vi "GetShooterRefs.vi"(8 "error in (no error)":errorcluster) -> (0 "error out":errorcluster, 3 "cluster out":T17={"Shooter Ratchet"={"DevStatus"={"status"=FALSE, "code"=0, "source"=""}, "Solenoid Module"=enum."Solenoid Module 1", "Forward Solenoid Channel"=enum."Solenoid 1", "Reverse Solenoid Channel"=enum."Solenoid 1"}, "Shooter Limit"={"DevStatus"={"status"=FALSE, "code"=0, "source"=""}, "DIO Channel"=enum."DIO 1", "Digital Module"=enum."Digital Module 1"}, "Shooter Dog"={"DevStatus"={"status"=FALSE, "code"=0, "source"=""}, "Solenoid Module"=enum."Solenoid Module 1", "Forward Solenoid Channel"=enum."Solenoid 1", "Reverse Solenoid Channel"=enum."Solenoid 1"}, "Wipers"={"DevStatus"={"status"=FALSE, "code"=0, "source"=""}, "Solenoid Module"=enum."Solenoid Module 1", "Forward Solenoid Channel"=enum."Solenoid 1", "Reverse Solenoid Channel"=enum."Solenoid 1"}, "Winch"={"DeviceStatus"={"status"=FALSE, "code"=0, "source"=""}, "Type"=enum."PWM", "PWM"={"Digital Module"=enum."Digital Module 1", "PWM Channel"=enum."PWM 1", "DeadBand"={"Name"="", "maxPositivePwm"=0, "minPositivePwm"=0, "centerPwm"=0, "maxNegativePwm"=0, "minNegativePwm"=0, "angularRange"=0}}, "CAN"={"Device Number"=0, "Control Mode"=enum."Percent VBus", "Semaphore"=refnum, "Max Vout"=0.0}, "Invert"=FALSE, "TransformRef"=refnum, "InvTransformRef"=refnum}, "Hall"={"DevStatus"={"status"=FALSE, "code"=0, "source"=""}, "DIO Channel"=enum."Invalid", "Digital Module"=enum."Digital Module 1"}, "Catch"={"DevStatus"={"status"=FALSE, "code"=0, "source"=""}, "Solenoid Module"=enum."Solenoid Module 1", "Forward Solenoid Channel"=enum."Invalid", "Reverse Solenoid Channel"=enum."Invalid"}, "Compressor"={"DevStatus"={"status"=FALSE, "code"=0, "source"=""}, "DigitalInputDevRef"={"DevStatus"={"status"=FALSE, "code"=0, "source"=""}, "DIO Channel"=enum."DIO 1", "Digital Module"=enum."Digital Module 1"}, "RelayDevRef"={"DevStatus"={"status"=FALSE, "code"=0, "source"=""}, "Relay Channel"=enum."Invalid", "Digital Module"=enum."Digital Module 1", "Relay Direction"=enum."Both directions"}}})   [LabVIEW 2013]
uses:
  <vilib>/Rock Robotics/WPI/Solenoid/WPI_SolenoidDevRef.ctl
  <vilib>/Rock Robotics/SystemInterfaces/Typedef/FPGA_TypedefSolenoidModule.ctl
  <vilib>/Rock Robotics/WPI/Solenoid/WPI_SolenoidChannel.ctl
  <vilib>/Rock Robotics/WPI/DigitalInput/WPI_DigitalInputDevRef.ctl
  <vilib>/Rock Robotics/SystemInterfaces/DIO/FPGA_DIOChannel.ctl
  <vilib>/Rock Robotics/SystemInterfaces/Typedef/FPGA_TypedefDigitalModule.ctl
  <vilib>/Rock Robotics/WPI/MotorControl/WPI_MotorControlDeviceRef.ctl
  <vilib>/Rock Robotics/SystemInterfaces/DIO/FPGA_DIOPWMChannel.ctl
  <vilib>/Rock Robotics/WPI/PWM/WPI_PWMDeadband.ctl
  <vilib>/Rock Robotics/WPI/CAN/Jaguar/SubVIs/WPI_CANJaguar_ControlMode.ctl
  <vilib>/Rock Robotics/WPI/PWM/WPI_PWMTransform_ConPane.ctl
  <vilib>/Rock Robotics/WPI/Compressor/WPI_CompressorDevRef.ctl
  <vilib>/Rock Robotics/WPI/Relay/WPI_RelayDevRef.ctl
  <vilib>/Rock Robotics/SystemInterfaces/DIO/FPGA_DIORelayChannel.ctl
  <vilib>/Rock Robotics/WPI/Relay/WPI_RelayDirection.ctl
panel:
  in  "cluster in":T17={"Shooter Ratchet"={"DevStatus"={"status"=FALSE, "code"=0, "source"=""}, "Solenoid Module"=enum."Solenoid Module 1", "Forward Solenoid Channel"=enum."Solenoid 1", "Reverse Solenoid Channel"=enum."Solenoid 1"}, "Shooter Limit"={"DevStatus"={"status"=FALSE, "code"=0, "source"=""}, "DIO Channel"=enum."DIO 1", "Digital Module"=enum."Digital Module 1"}, "Shooter Dog"={"DevStatus"={"status"=FALSE, "code"=0, "source"=""}, "Solenoid Module"=enum."Solenoid Module 1", "Forward Solenoid Channel"=enum."Solenoid 1", "Reverse Solenoid Channel"=enum."Solenoid 1"}, "Wipers"={"DevStatus"={"status"=FALSE, "code"=0, "source"=""}, "Solenoid Module"=enum."Solenoid Module 1", "Forward Solenoid Channel"=enum."Solenoid 1", "Reverse Solenoid Channel"=enum."Solenoid 1"}, "Winch"={"DeviceStatus"={"status"=FALSE, "code"=0, "source"=""}, "Type"=enum."PWM", "PWM"={"Digital Module"=enum."Digital Module 1", "PWM Channel"=enum."PWM 1", "DeadBand"={"Name"="", "maxPositivePwm"=0, "minPositivePwm"=0, "centerPwm"=0, "maxNegativePwm"=0, "minNegativePwm"=0, "angularRange"=0}}, "CAN"={"Device Number"=0, "Control Mode"=enum."Percent VBus", "Semaphore"=refnum, "Max Vout"=0.0}, "Invert"=FALSE, "TransformRef"=refnum, "InvTransformRef"=refnum}, "Hall"={"DevStatus"={"status"=FALSE, "code"=0, "source"=""}, "DIO Channel"=enum."Invalid", "Digital Module"=enum."Digital Module 1"}, "Catch"={"DevStatus"={"status"=FALSE, "code"=0, "source"=""}, "Solenoid Module"=enum."Solenoid Module 1", "Forward Solenoid Channel"=enum."Invalid", "Reverse Solenoid Channel"=enum."Invalid"}, "Compressor"={"DevStatus"={"status"=FALSE, "code"=0, "source"=""}, "DigitalInputDevRef"={"DevStatus"={"status"=FALSE, "code"=0, "source"=""}, "DIO Channel"=enum."DIO 1", "Digital Module"=enum."Digital Module 1"}, "RelayDevRef"={"DevStatus"={"status"=FALSE, "code"=0, "source"=""}, "Relay Channel"=enum."Invalid", "Digital Module"=enum."Digital Module 1", "Relay Direction"=enum."Both directions"}}}
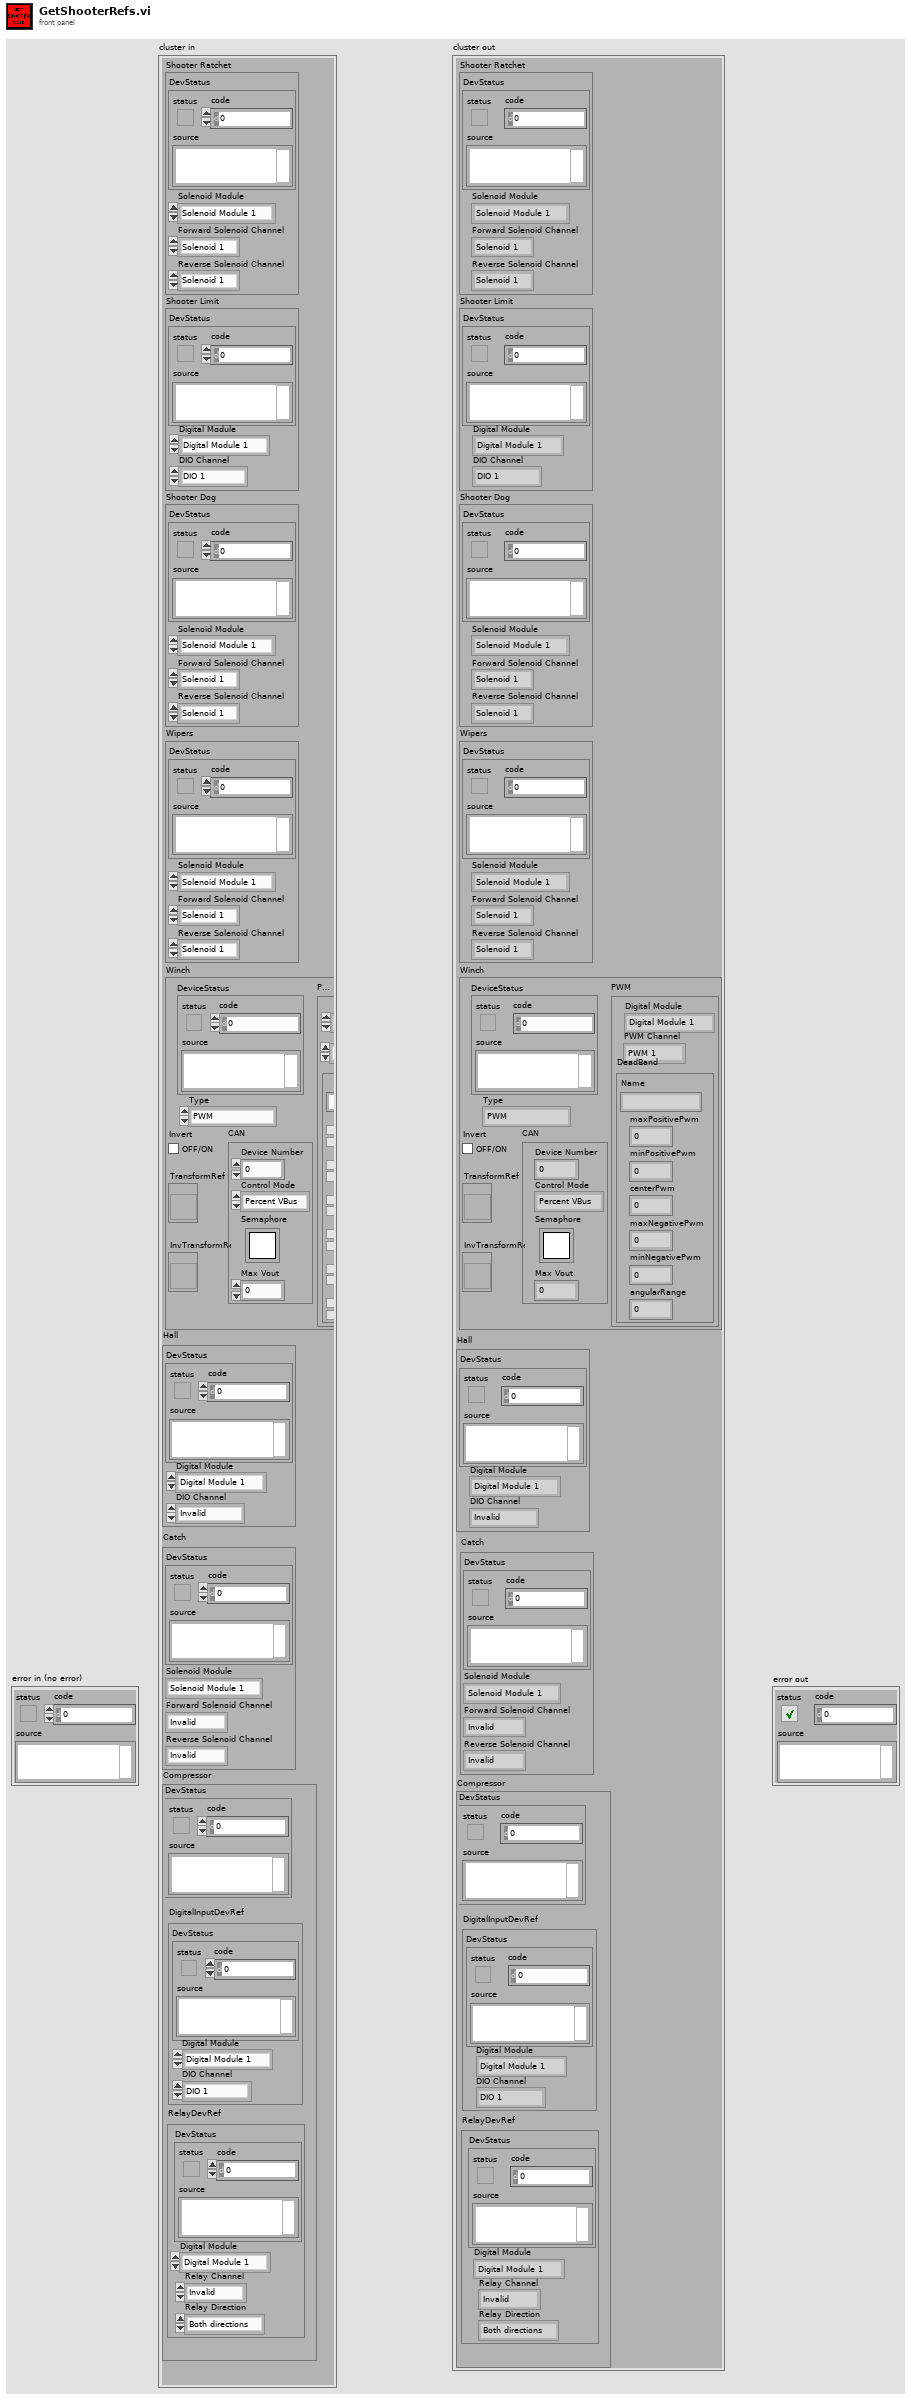
[diagram p1: front panel]
types:
  T1 = typedef "WPI_SolenoidDevRef.ctl" = cluster{"DevStatus":errorcluster, "Solenoid Module":T2, "Forward Solenoid Channel":T3, "Reverse Solenoid Channel":T3}
  T2 = typedef "FPGA_TypedefSolenoidModule.ctl" = enum16{"Solenoid Module 1", "Solenoid Module 2"}
  T3 = typedef "WPI_SolenoidChannel.ctl" = enum8{"Solenoid 1", "Solenoid 2", "Solenoid 3", "Solenoid 4", "Solenoid 5", "Solenoid 6", "Solenoid 7", "Solenoid 8", "Invalid"}
  T4 = typedef "WPI_DigitalInputDevRef.ctl" = cluster{"DevStatus":errorcluster, "DIO Channel":T5, "Digital Module":T6}
  T5 = typedef "FPGA_DIOChannel.ctl" = enum8{"DIO 1", "DIO 2", "DIO 3", "DIO 4", "DIO 5", "DIO 6", "DIO 7", "DIO 8", "DIO 9", "DIO 10", "DIO 11", "DIO 12", "DIO 13", "DIO 14", "Invalid"}
  T6 = typedef "FPGA_TypedefDigitalModule.ctl" = enum16{"Digital Module 1", "Digital Module 2"}
  T7 = typedef "WPI_MotorControlDeviceRef.ctl" = cluster{"DeviceStatus":errorcluster, "Type":enum16{"PWM", "CAN"}, "PWM":cluster{"Digital Module":T6, "PWM Channel":T8, "DeadBand":T9}, "CAN":cluster{"Device Number":u8, "Control Mode":T10, "Semaphore":T11, "Max Vout":dbl}, "Invert":bool, "TransformRef":T12, "InvTransformRef":T12}
  T8 = typedef "FPGA_DIOPWMChannel.ctl" = enum8{"PWM 1", "PWM 2", "PWM 3", "PWM 4", "PWM 5", "PWM 6", "PWM 7", "PWM 8", "PWM 9", "PWM 10", "Invalid"}
  T9 = typedef "WPI_PWMDeadband.ctl" = cluster{"Name":string, "maxPositivePwm":i32, "minPositivePwm":i32, "centerPwm":i32, "maxNegativePwm":i32, "minNegativePwm":i32, "angularRange":u16}
  T10 = typedef "WPI_CANJaguar_ControlMode.ctl" = enum8{"Percent VBus", "Current", "Speed", "Position", "Voltage"}
  T11 = typedef "Semaphore RefNum" = refnum<k1>
  T12 = typedef "WPI_PWMTransform_ConPane.ctl" = refnum<vi>
  T13 = typedef "WPI_CompressorDevRef.ctl" = cluster{"DevStatus":errorcluster, "DigitalInputDevRef":T4, "RelayDevRef":T14}
  T14 = typedef "WPI_RelayDevRef.ctl" = cluster{"DevStatus":errorcluster, "Relay Channel":T15, "Digital Module":T6, "Relay Direction":T16}
  T15 = typedef "FPGA_DIORelayChannel.ctl" = enum8{"Relay 1", "Relay 2", "Relay 3", "Relay 4", "Relay 5", "Relay 6", "Relay 7", "Relay 8", "Invalid"}
  T16 = typedef "WPI_RelayDirection.ctl" = enum16{"Both directions", "Forward only", "Reverse only"}
  T17 = cluster{"Shooter Ratchet":T1, "Shooter Limit":T4, "Shooter Dog":T1, "Wipers":T1, "Winch":T7, "Hall":T4, "Catch":T1, "Compressor":T13}
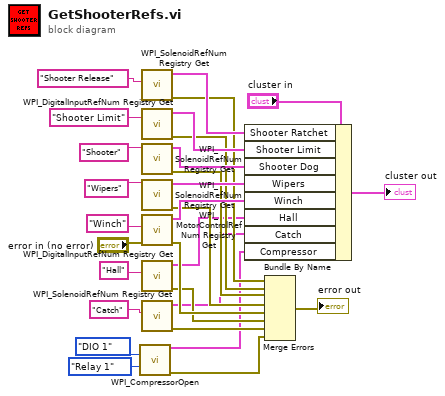
[diagram p0: block diagram]
diagram:
  n1 = call <vilib>:"WPI_CompressorOpen.vi"("Pressure Switch DIO Channel"=FPGA_DIOChannel."DIO 1", "Relay Channel"=FPGA_DIORelayChannel."Relay 1") -> ("CompressorDevRef"=w1:T13, "error out"=w2:errorcluster)  [unwired: 12 in]
  n2 = call <vilib>:"WPI_SolenoidRefNum Registry Get.vi"("refnum name"="Shooter Release") -> ("error out"=w17:errorcluster, "SolenoidDevRef"=w23:T1)  [unwired: 9 in]
  n3 = call <vilib>:"WPI_DigitalInputRefNum Registry Get.vi"("refnum name"="Shooter Limit") -> ("error out"=w16:errorcluster, "DigitalInputDevRef"=w24:T4)  [unwired: 9 in]
  n4 = call <vilib>:"WPI_SolenoidRefNum Registry Get.vi"("refnum name"="Shooter") -> ("error out"=w15:errorcluster, "SolenoidDevRef"=w25:T1)  [unwired: 9 in]
  n5 = call <vilib>:"WPI_SolenoidRefNum Registry Get.vi"("refnum name"="Wipers") -> ("error out"=w14:errorcluster, "SolenoidDevRef"=w26:T1)  [unwired: 9 in]
  n6 = call <vilib>:"WPI_MotorControlRefNum Registry Get.vi"("error in (no error)"="error in (no error)", "refnum name"="Winch") -> ("error out"=w13:errorcluster, "MotorControlDevRef"=w27:T7)  [unwired: 8 in]
  n7 = call <vilib>:"WPI_DigitalInputRefNum Registry Get.vi"("refnum name"="Hall") -> ("error out"=w8:errorcluster, "DigitalInputDevRef"=w9:T4)  [unwired: 9 in]
  n8 = call <vilib>:"WPI_SolenoidRefNum Registry Get.vi"("refnum name"="Catch") -> ("error out"=w6:errorcluster, "SolenoidDevRef"=w5:T1)  [unwired: 9 in]
  n9 = Bundle By Name(cluster="cluster in", "Shooter Ratchet"=w23, "Shooter Limit"=w24, "Shooter Dog"=w25, "Wipers"=w26, "Winch"=w27, "Hall"=w9, "Catch"=w5, "Compressor"=w1) -> (→"cluster out":T17)
  n10 = Merge Errors(w17, w16, w15, w14, w13, w8, w6, w2) -> (→"error out":errorcluster)
